vi "uMsg Send Reply.vi"(8 "error in (no error)":errorcluster, 10 "Reply Data":refnum<class "uData.lvclass">, 11 "Original Msg":refnum<class "uMsg.lvclass">) -> (0 "error out":errorcluster)   [LabVIEW 2021, in "uFramework.lvlib" / "uMsg.lvclass"]
doc: "Send a reply message to the original message sender.\nThis sends a reply regardless of the error-in state, This to prevent external actors from waiting unnecessarily. The error in value only impacts the ACK/NAK status in the reply message."
uses:
  uMsg.lvclass
  Bin/uData.lvlibp/uData.lvclass
  uMsg.lvclass/uMsg.ctl
  uTransport/uTransport.lvclass
  uMsg Update Timestamp.vi
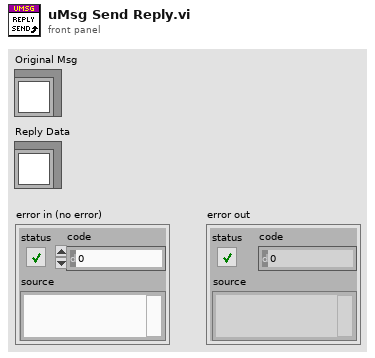
[diagram p1: front panel]
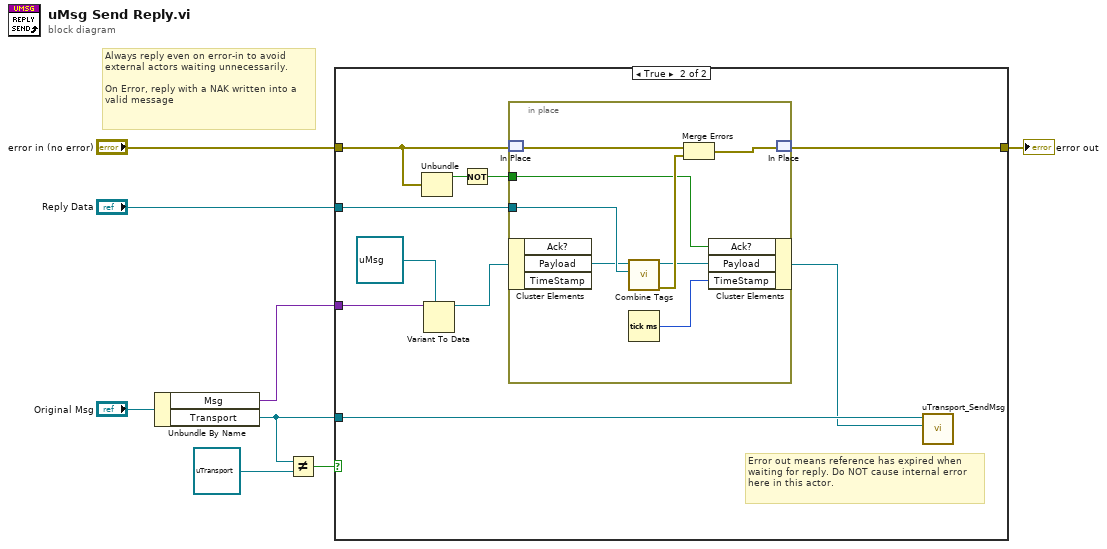
[diagram p0: block diagram]
diagram:
  # "Always reply even on error-in to avoid external actors waiting unnecessarily.\n\nOn Error, reply with a NAK written into a valid message"
  n1 = Unbundle By Name("Original Msg") -> ("Msg"=w8:variant, "Transport"=w3:refnum<class "uTransport.lvclass">)
  n2 = Not Equal?(x=w3, y=refnum<class "uTransport.lvclass"> refnum) -> (x != y?=w1:bool)
  n3 = case shown="True" w1 {
    tunnel: w8 -> [_ w16]
    tunnel: "Reply Data" -> [_ w10]
    tunnel: "error in (no error)" -> [w9 w15]
    tunnel: [w9 w14] -> w5
    tunnel: w3 -> [_ w13]
    frame False {
      # "Avoid unnecessary dynamic dispatch overhead when the reply address is not provided"
    }
    frame True {
      # "Error out means reference has expired when waiting for reply. Do NOT cause internal error here in this actor."
      n4 = Unbundle(w15) -> ("status"=w19:bool)  [unwired: 2 out]
      n5 = Variant To Data(type=refnum<class "uMsg.lvclass"> refnum ("uMsg.lvclass"), Variant=w16) -> (data=w12:refnum<class "uMsg.lvclass">)  [unwired: 1 in, 1 out]
      n6 = Not(x=w19) -> (.not. x?=w17:bool)
      n7 = in-place {
        in-place-border: w17 -> [w26]
        in-place-border: w10 -> [w21]
        n8 = in-place-match #1(w15) -> (w25:errorcluster)
        n9 = in-place-cluster #2(w12) -> ("Payload"=w20:refnum<class "uData.lvclass">)  [unwired: 2 out]
        n10 = call "Combine Tags.vi"("Appended uData"=w21, "Base uData"=w20) -> ("error out"=w27:errorcluster, "Combined uData"=w22:refnum<class "uData.lvclass">)  [unwired: 7 in, 1 out]
        n11 = Tick Count (ms)() -> (millisecond timer value=w23:u32)
        n12 = Merge Errors(w25, w27) -> (w24:errorcluster)
        n13 = in-place-cluster #2("Ack?"=w26, "Payload"=w22, "TimeStamp"=w23) -> (w11:refnum<class "uMsg.lvclass">)
        n14 = in-place-match #1(w24) -> (w14:errorcluster)
      }
      n15 = call "uTransport_SendMsg.vi"("Msg"=w11, "uTransport in"=w13) -> ()  [unwired: 8 in, 2 out]
    }
  }
  "error out" <- w5
